vi "DO Convert Data to JSON string.vi"(8 "error in":errorcluster, 10 "DO Config Data":T1, 11 "Data In":bool[](array[boolean])) -> (0 "error out":errorcluster, 3 "JSON String":string)   [LabVIEW 2024]
uses:
  Host-DQMH/Configuration/DO Channel's.ctl
  Host-Control's/TCP Tx-Rx cluster.ctl
  <vilib>/addons/_JKI.lib/Serialization/JSON/JKI JSON Serialization.lvlib
  RT-DQMH-Module's/RT-TDMS-Logging/RT-TDMS-Logging.lvlib
  Host-DQMH/Configuration/Configuration.lvlib
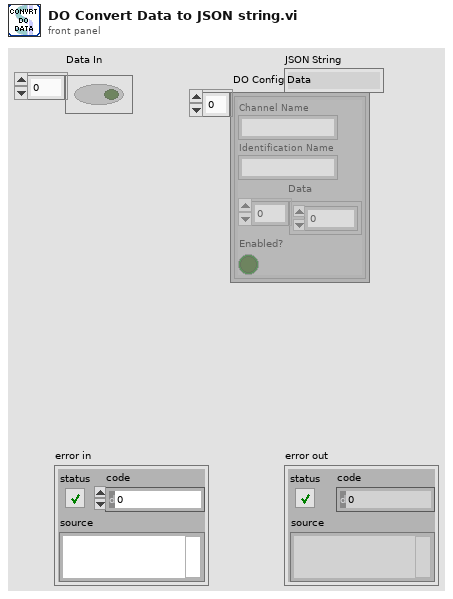
[diagram p1: front panel]
types:
  T1 = typedef "Configuration.lvlib/DO Channel's.ctl" = cluster{"Channel Name":string, "Identification Name":string, "Data":u8[], "Enabled?":bool}[]
  T2 = typedef "TCP Tx-Rx cluster.ctl" = cluster{"Interface":string, "Command":string, "SubCmd":string, "Data":variant}
  T3 = cluster{"Channels":string[], "Data":i16[], "Time":string}
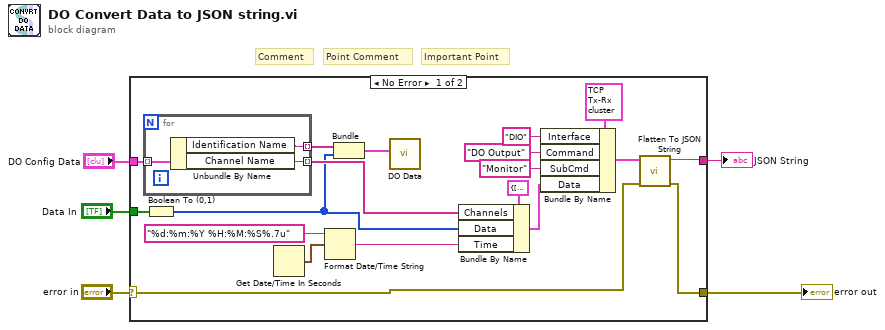
[diagram p0: block diagram]
diagram:
  # "Important Point"
  # "Point Comment"
  # "Comment"
  n1 = case shown="No Error" "error in" {
    selector: "error in" -> [w7 w28]
    tunnel: [w10 w28] -> w5
    tunnel: "Data In" -> [w24 _]
    tunnel: [w11 _] -> w2
    tunnel: "DO Config Data" -> [w23 _]
    frame No Error {
      n2 = for {
        tunnel: w23 -> [w27] mode=indexing
        tunnel: [w26] -> w15 mode=indexing
        tunnel: [w25] -> w9 mode=indexing
        n3 = Unbundle By Name(w27) -> ("Identification Name"=w25:string, "Channel Name"=w26:string)
      }
      n4 = Boolean To (0,1)(Boolean=w24) -> (0, 1=w8:i16[])
      n5 = Get Date/Time In Seconds() -> (seconds since 1Jan1904=w13:timestamp)
      n6 = Format Date/Time String(time format string (%c)="%d:%m:%Y %H:%M:%S%.7u", seconds (now)=w13) -> (date/time string=w16:string)  [unwired: 1 in]
      n7 = Bundle(w9, w8) -> (w6:cluster{string[], i16[]})  [unwired: 1 in]
      n8 = call "DO Data.vi"("DO Data"=w6) -> ()  [unwired: 10 in, 1 out]
      n9 = Bundle By Name(cluster=T3 {"Channels"=[], "Data"=[], "Time"=""}, "Channels"=w15, "Data"=w8, "Time"=w16) -> (w14:T3)
      n10 = Bundle By Name(cluster=T2 {"Interface"="CPU", "Command"="CPU Info", "SubCmd"="Monitor", "Data"=variant} ("TCP Tx-Rx Cluster"), "Interface"="DIO", "Command"="DO Output", "SubCmd"="Monitor" ("Sub Cmd"), "Data"=w14) -> (w12:T2)
      n11 = call <vilib>:"Flatten To JSON String.vi"("error in"=w7, "Variant"=w12) -> ("error out"=w10:errorcluster, "JSON String"=w11:string)  [unwired: 8 in]
    }
    frame Error {
    }
  }
  "error out" <- w5
  "JSON String" <- w2
